vi "postPro.vi"() -> ()   [LabVIEW 2018]
panel:
  in  "Threshold":dbl=1.75
  in  "Method A (Left), Method B (Right)":bool
  in  "Tab Control":enum32{"Pull Method A", "Pull Method B"}(tab)
  in  "Number of Files":i32=80
  in  "Number of Heights":i32=4
  out "In Folder":string
  out "Probe No":string
  in  "MET Data.csv":path
  in  "Data Path":string
  in  "ESDU Path":path=path "" caption="start path"
  out "Output Data":string[][](array[string])
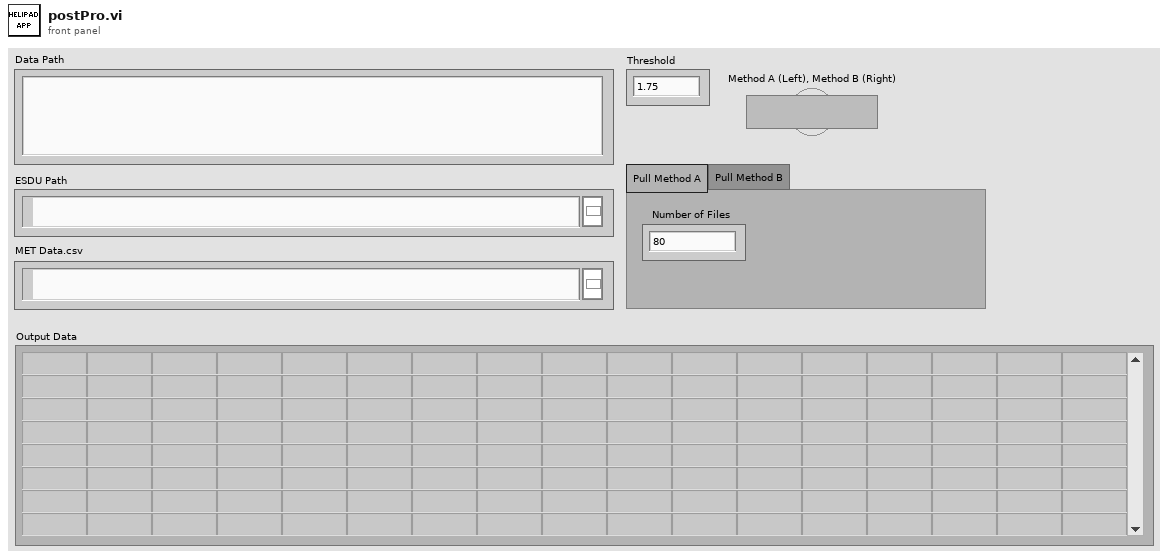
[diagram p1: front panel]
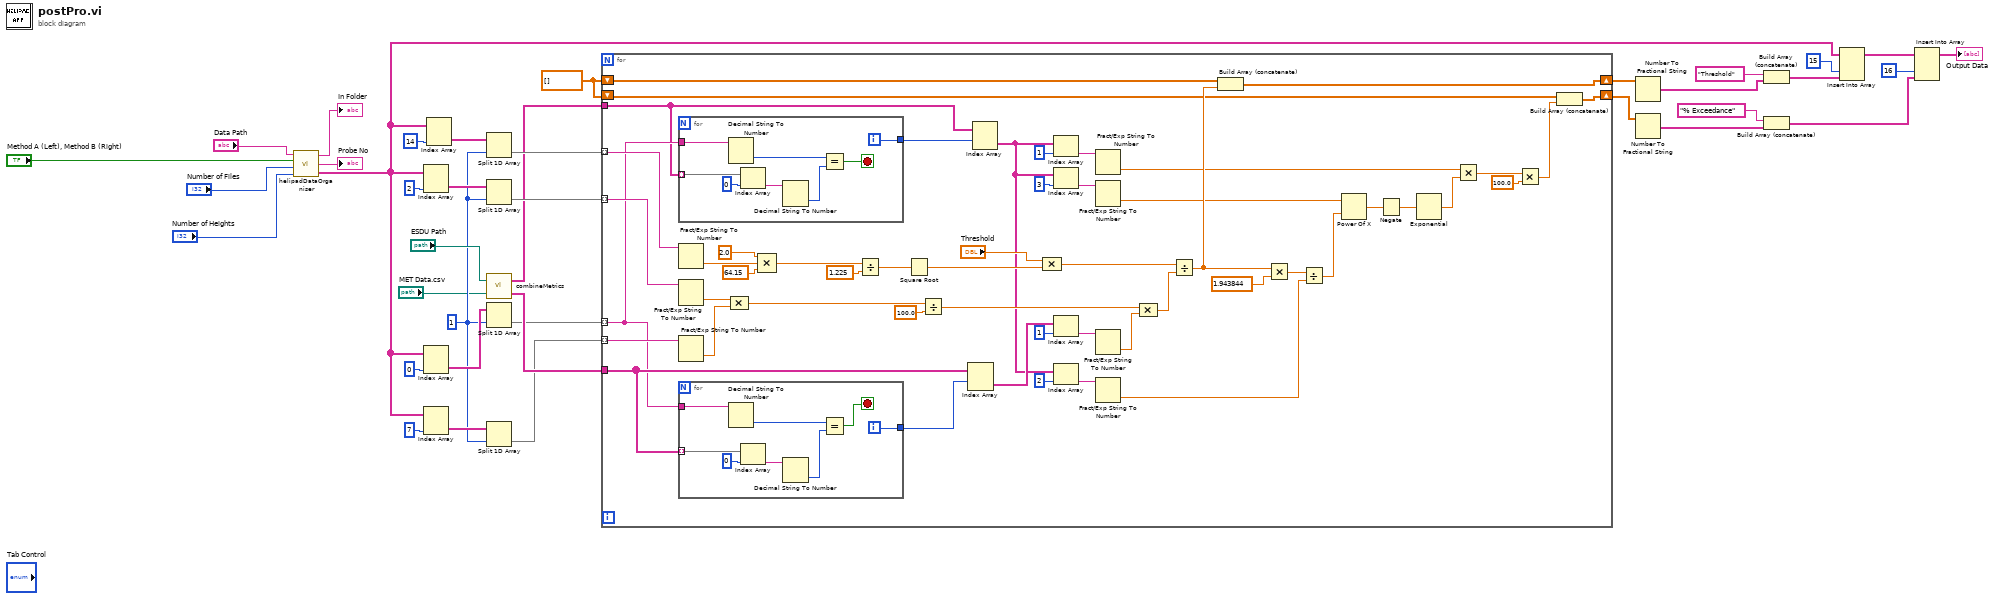
[diagram p0: block diagram]
diagram:
  w17 = 1 ("index")
  w15 = dbl[] []
  n1 = call "helipadDataOrganiser.vi"("Number of Heights"="Number of Heights", "Number of Files"="Number of Files", "Method A (Left), Method B (Right)"="Method A (Left), Method B (Right)", "Data Path"="Data Path") -> ("Output Data"=w30:string[][], "Probe No"=→"Probe No":string, "In Folder"=→"In Folder":string)
  n2 = Index Array(array=w30, index (col)=2 ("disabled index (col)")) -> (element=w22:string[])  [unwired: 1 in]
  n3 = Index Array(array=w30, index (col)=0 ("disabled index (col)")) -> (element=w18:string[])  [unwired: 1 in]
  n4 = Index Array(array=w30, index (col)=7 ("disabled index (col)")) -> (element=w20:string[])  [unwired: 1 in]
  n5 = Index Array(array=w30, index (col)=14 ("disabled index (col)")) -> (element=w24:string[])  [unwired: 1 in]
  n6 = Split 1D Array(array=w24, index=w17) -> (second subarray=w23:string[])  [unwired: 1 out]
  n7 = Split 1D Array(array=w22, index=w17) -> (second subarray=w21:string[])  [unwired: 1 out]
  n8 = call "combineMetrics.vi"("MET Data.csv"="MET Data.csv", "ESDU Path"="ESDU Path") -> ("ESDU Mean Factors"=w25:string[][], "Annual Met Data"=w6:string[][])
  n9 = Split 1D Array(array=w18, index=w17) -> (second subarray=w16:string[])  [unwired: 1 out]
  n10 = Split 1D Array(array=w20, index=w17) -> (second subarray=w19:string[])  [unwired: 1 out]
  n11 = for {
    tunnel: w23 -> [w86] mode=indexing
    shift-right: [w81] -> w31
    shift-left: w15 -> [w80]
    tunnel: w21 -> [w78] mode=indexing
    tunnel: w25 -> [w69]
    tunnel: w16 -> [w50] mode=indexing
    tunnel: w19 -> [w67] mode=indexing
    shift-right: [w60] -> w14
    shift-left: w15 -> [w59]
    tunnel: w6 -> [w49]
    n12 = for {
      tunnel: w50 -> [w93]
      tunnel: w49 -> [w95] mode=indexing
      tunnel: [w89] -> w48
      i -> [w89]
      stop <- w90 stop-if-true
      n13 = Decimal String To Number(string=w93) -> (number=w92:i32)  [unwired: 2 in, 1 out]
      n14 = Index Array(array=w95, index=0) -> (element=w91:string)
      n15 = Decimal String To Number(string=w91) -> (number=w94:i32)  [unwired: 2 in, 1 out]
      n16 = Equal?(x=w92, y=w94) -> (x = y?=w90:bool)
    }
    n17 = Fract/Exp String To Number(string=w86) -> (number=w87:dbl)  [unwired: 3 in, 1 out]
    n18 = Fract/Exp String To Number(string=w78) -> (number=w77:dbl)  [unwired: 3 in, 1 out]
    n19 = Fract/Exp String To Number(string=w67) -> (number=w76:dbl)  [unwired: 3 in, 1 out]
    n20 = for {
      tunnel: w50 -> [w101]
      tunnel: w69 -> [w103] mode=indexing
      tunnel: [w97] -> w68
      i -> [w97]
      stop <- w98 stop-if-true
      n21 = Decimal String To Number(string=w101) -> (number=w100:i32)  [unwired: 2 in, 1 out]
      n22 = Index Array(array=w103, index=0) -> (element=w99:string)
      n23 = Decimal String To Number(string=w99) -> (number=w102:i32)  [unwired: 2 in, 1 out]
      n24 = Equal?(x=w100, y=w102) -> (x = y?=w98:bool)
    }
    n25 = Compound Arithmetic op=MULTIPLY(w77, w76) -> (w75:dbl)
    n26 = Compound Arithmetic op=MULTIPLY(2.0, w87, 64.15 ("value")) -> (w84:dbl)
    n27 = Divide(x=w84, y=1.225) -> (x/y=w82:dbl)
    n28 = Square Root(x=w82) -> (sqrt(x)=w79:dbl)
    n29 = Divide(x=w75, y=100.0) -> (x/y=w71:dbl)
    n30 = Index Array(array=w69, index (row)=w68) -> (element=w70:string[])  [unwired: 1 in]
    n31 = Index Array(array=w49, index (row)=w48) -> (element=w38:string[])  [unwired: 1 in]
    n32 = Compound Arithmetic op=MULTIPLY("Threshold", w79) -> (w73:dbl)
    n33 = Index Array(array=w38, index=1) -> (element=w41:string)
    n34 = Index Array(array=w38, index=3) -> (element=w39:string)
    n35 = Index Array(array=w70, index=1) -> (element=w42:string)
    n36 = Index Array(array=w38, index=2) -> (element=w40:string)
    n37 = Fract/Exp String To Number(string=w41) -> (number=w54:dbl)  [unwired: 3 in, 1 out]
    n38 = Fract/Exp String To Number(string=w39) -> (number=w52:dbl)  [unwired: 3 in, 1 out]
    n39 = Fract/Exp String To Number(string=w42) -> (number=w47:dbl)  [unwired: 3 in, 1 out]
    n40 = Fract/Exp String To Number(string=w40) -> (number=w53:dbl)  [unwired: 3 in, 1 out]
    n41 = Compound Arithmetic op=MULTIPLY(w71, w47) -> (w72:dbl)
    n42 = Divide(x=w73, y=w72) -> (x/y=w66:dbl)
    n43 = Build Array (concatenate)(w80, w66) -> (w81:dbl[])
    n44 = Multiply(x=w66, y=1.943844) -> (x*y=w64:dbl)
    n45 = Divide(x=w64, y=w53) -> (x/y=w55:dbl)
    n46 = Power Of X(1:w55, 2:w52) -> (0:w63:dbl)
    n47 = Negate(x=w63) -> (-x=w62:dbl)
    n48 = Exponential(1:w62) -> (0:w61:dbl)
    n49 = Multiply(x=w54, y=w61) -> (x*y=w58:dbl)
    n50 = Multiply(x=w58, y=100.0) -> (x*y=w56:dbl)
    n51 = Build Array (concatenate)(w59, w56) -> (w60:dbl[])
  }
  n52 = Number To Fractional String(number=w31) -> (F-format string=w27:string[])  [unwired: 3 in]
  n53 = Number To Fractional String(number=w14) -> (F-format string=w12:string[])  [unwired: 3 in]
  n54 = Build Array (concatenate)("Threshold", w27) -> (w26:string[])
  n55 = Build Array (concatenate)("% Exceedance", w12) -> (w10:string[])
  n56 = Insert Into Array(array=w30, index (col)=15 ("disabled index (col)"), new element=w26) -> (w13:string[][])  [unwired: 1 in]
  n57 = Insert Into Array(array=w13, index (col)=16 ("disabled index (col)"), new element=w10) -> (→"Output Data":string[][])  [unwired: 1 in]
